vi "Robot Global Data.vi"() -> ()   [LabVIEW 2017]
doc: "This global VI can contain as many global variables as you need. Place a control on the panel, give it a good name. To read or write to it from a VI, drag the icon to the diagram of that VI. You can also drag from the project. Click on the node to change which global you access. You shouldn't have multiple locations writing to a global or it will cause a race-condition."
uses:
  <vilib>/Rock Robotics/WPI/Camera/WPI_CameraImageSize.ctl
  <vilib>/Rock Robotics/WPI/DriverStation/WPI_DriverStationRobotMode2.ctl
panel:
  in  "DriveTrainShifter":bool
  in  "LifterShifter":bool
  out "Gyro-Raw":dbl
  out "Gyro-FusedHeading":dbl
  in  "Reset-LiftEncoder":bool
  in  "Reset-DriveEncoder":bool
  in  "Reset-Gyro":bool
  in  "Arm":bool
  in  "Gripper":bool
  out "RangeFinder":dbl
  in  "AnglePIDGains":cluster{"P":dbl, "I":dbl, "D":dbl}={"P"=0.05, "I"=0.0035, "D"=0.001}
  in  "Reset-All":bool
  out "MatchInfo":string
  out "LifterEncoder":dbl
  out "CurrentDirection":dbl
  out "DriveLeft":dbl
  out "DriveRight":dbl
  out "Gyro":dbl
  out "RightEncoder":dbl
  out "LeftEncoder":dbl
  in  "Robot Mode":T1
  in  "image size":T2=enum."320x240"
  in  "Enable Vision":bool
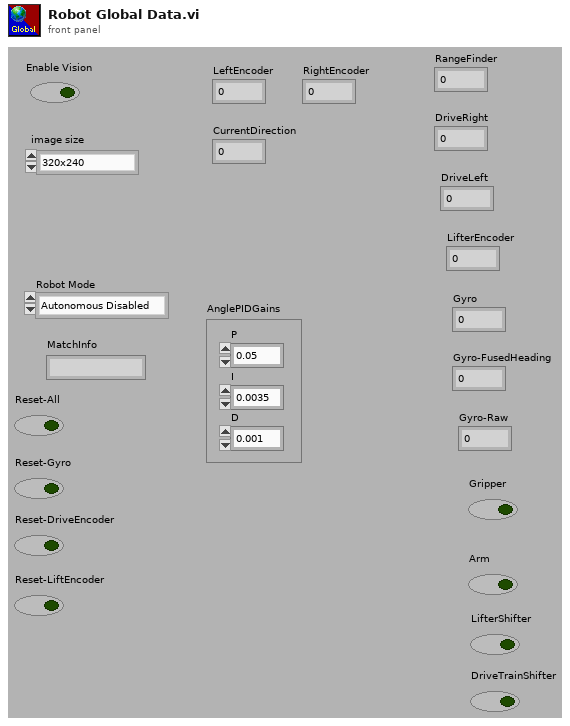
[diagram p1: front panel]
types:
  T1 = typedef "WPI_DriverStationRobotMode2.ctl" = enum16{"Autonomous Disabled", "Autonomous Enabled", "Teleop Disabled", "Teleop Enabled", "Disconnected", "Finish", "Test Disabled", "Test Enabled", "Emergency Stopped"}
  T2 = typedef "WPI_CameraImageSize.ctl" = enum16{"640x480", "320x240", "160x120", "Custom"}
diagram:
